vi "Initiate Updates.vi"(8 "error in (no error)":errorcluster, 11 "IDialogBox In":refnum<class "IDialogBox.lvclass">) -> (0 "error out":errorcluster, 3 "IDialogBox Out":refnum<class "IDialogBox.lvclass">)   [LabVIEW 2018, in "MVA Framework.lvlib" / "IDialogBox.lvlib" / "IDialogBox.lvclass"]
doc: "初始化更新"
uses:
  IDialogBox.lvclass
  modules/mva-viewable/Source/IViewable/IViewable/IViewable.lvclass
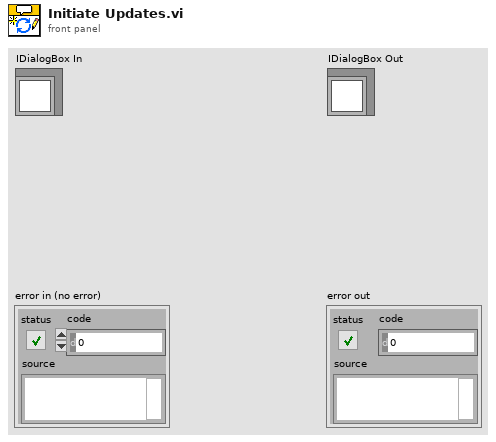
[diagram p1: front panel]
types:
  T1 = enum32{"Invalid", "Standard", "Closed", "Hidden", "Minimized", "Maximized"}
  T2 = enum32{"Invalid", "Default", "Floating", "Floating/Auto-Hide", "Modal"}
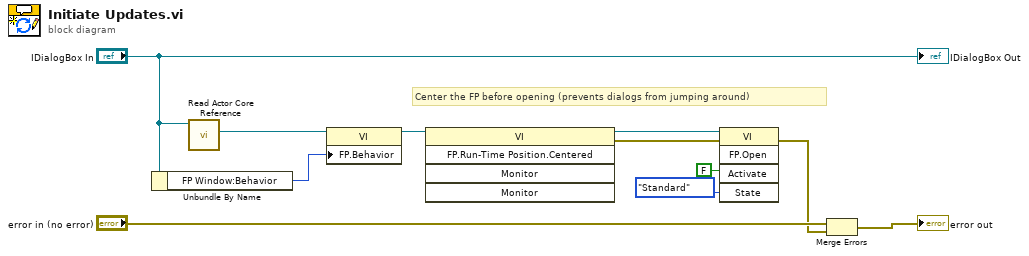
[diagram p0: block diagram]
diagram:
  # "Center the FP before opening (prevents dialogs from jumping around)"
  n1 = Unbundle By Name("IDialogBox In") -> ("FP Window:Behavior"=w1:T2)
  n2 = call "Read Actor Core Reference.vi"("IViewable In"="IDialogBox In") -> ("Actor Core Refnum"=w4:refnum<vi>)  [unwired: 9 in, 1 out]
  n3 = property class="VI"(reference=w4, "FP.Behavior"=w1) -> (reference out=w3:refnum<vi>)  [unwired: 1 in, 1 out]
  n4 = invoke class="VI" method="FP.Run-Time Position.Centered"(reference=w3) -> (reference out=w7:refnum<vi>, error out=w9:errorcluster)  [unwired: 4 in, 3 out]
  n5 = invoke class="VI" method="FP.Open"(reference=w7, error in=w9, "Activate"=FALSE ("Activate?"), "State"=T1."Standard") -> (error out=w8:errorcluster)  [unwired: 1 in, 4 out]
  n6 = Merge Errors("error in (no error)", w8) -> (→"error out":errorcluster)
  "IDialogBox Out" <- "IDialogBox In"
